vi "CP FES Thresholding.vi"(3 "CP FES Walking Data":T1={"Subject"=0, "Subject Parameter File"=path "", "Subject Parameters"={"Subject"=0, "Left GPD Params"={"% Cycle Delay"=75.0, "Min % Cycle LR to ISw "=55.0, "Min % Cycle LR to MSw"=50.0, "Min % Cycle LR to TSw"=75.0, "Max % Cycle ISw to MSw"=10.0, "Min % Cycle TSw to LR"=2.5, "Max % Cycle TSw to LR"=75.0, "LR Min Gyro Z Threshold"=-0.3, "LR Min Gyro Z Width"=230.0, "ISw Peak Threshold"=0.6, "ISw Peak Width"=55.0, "TSw Valley Threshold"=-0.5, "TSw Valley Width (ms)"=55.0, "Max Cycle Time (s)"=1.3, "Mean Computation Window"=10.0, "CP subject?"=FALSE}, "Right GPD Params"={"% Cycle Delay"=75.0, "Min % Cycle LR to ISw "=55.0, "Min % Cycle LR to MSw"=50.0, "Min % Cycle LR to TSw"=75.0, "Max % Cycle ISw to MSw"=10.0, "Min % Cycle TSw to LR"=2.5, "Max % Cycle TSw to LR"=75.0, "LR Min Gyro Z Threshold"=-0.3, "LR Min Gyro Z Width"=230.0, "ISw Peak Threshold"=0.6, "ISw Peak Width"=55.0, "TSw Valley Threshold"=-0.5, "TSw Valley Width (ms)"=55.0, "Max Cycle Time (s)"=1.3, "Mean Computation Window"=10.0, "CP subject?"=FALSE}, "Left Stim Params"={"Stim Pattern Values"=[[enum."Full", enum."Half", enum."Off", enum."Off", enum."Off", enum."Off", enum."Half"], [enum."Full", enum."Off", enum."Off", enum."Off", enum."Off", enum."Half", enum."Half"], [enum."Half", enum."Full", enum."Off", enum."Full", enum."Off", enum."Off", enum."Full"], [enum."Half", enum."Off", enum."Off", enum."Half", enum."Full", enum."Full", enum."Full"], [enum."Off", enum."Full", enum."Half", enum."Half", enum."Off", enum."Off", enum."Off"]], "Pulse Duration"=[20, 200, 200, 200, 200], "Current"=[20, 20, 20, 20, 20]}, "Right Stim Params"={"Stim Pattern Values"=[[enum."Full", enum."Half", enum."Off", enum."Off", enum."Off", enum."Off", enum."Half"], [enum."Full", enum."Off", enum."Off", enum."Off", enum."Off", enum."Half", enum."Half"], [enum."Half", enum."Full", enum."Off", enum."Full", enum."Off", enum."Off", enum."Full"], [enum."Half", enum."Off", enum."Off", enum."Half", enum."Full", enum."Full", enum."Full"], [enum."Off", enum."Full", enum."Half", enum."Half", enum."Off", enum."Off", enum."Off"]], "Pulse Duration"=[200, 200, 200, 200, 200], "Current"=[200, 200, 200, 200, 200]}, "Left Train length"=[300, 300, 300, 300, 300], "Right Train length"=[300, 300, 300, 300, 300]}, "Current Interval Idx"=0, "Protocol"={"Active Interval"=[], "Protocol"=[{"Interval Type"=enum."Walk", "Duration"=20.0, " Mode"=enum."Stim", "Alt Period"=0.0}, {"Interval Type"=enum."Rest", "Duration"=20.0, " Mode"=enum."No Stim", "Alt Period"=0.0}, {"Interval Type"=enum."Walk", "Duration"=20.0, " Mode"=enum."Stim", "Alt Period"=0.0}, {"Interval Type"=enum."Rest", "Duration"=20.0, " Mode"=enum."No Stim", "Alt Period"=0.0}, {"Interval Type"=enum."Walk", "Duration"=20.0, " Mode"=enum."Stim", "Alt Period"=0.0}, {"Interval Type"=enum."Rest", "Duration"=20.0, " Mode"=enum."No Stim", "Alt Period"=0.0}, {"Interval Type"=enum."Walk", "Duration"=20.0, " Mode"=enum."Stim", "Alt Period"=0.0}, {"Interval Type"=enum."Rest", "Duration"=20.0, " Mode"=enum."No Stim", "Alt Period"=0.0}, {"Interval Type"=enum."Walk", "Duration"=20.0, " Mode"=enum."Alternating", "Alt Period"=0.0}]}, "Stim Protocol Log File"=path "", "APDM Init Cluster"={"Log Data"=TRUE, "Gyro Mode"="SIMULATE GYRO", "Left  OPAL ID"=0, "Right OPAL ID"=0, "Access Point ID"=0}, "Stimulators"=[]} {"Subject" items=["Subject 0", "Subject 1", "Subject 2", "Subject 3", "Subject 4", "Subject 5", "Subject 6", "Subject 7", "Subject 8", "Subject 9", "Subject 10", "Subject 11", "Subject 12", "Subject 13", "Subject 14", "Subject 15", "Subject 16", "Subject 17", "Subject 18", "Subject 19", "Subject 20", "Subject 21", "Subject 22", "Subject 23", "Subject 24", "Subject 25", "Subject 26", "Subject 27", "Subject 28", "Subject 29", "Subject 30", "Subject 31", "Subject 32", "Subject 33", "Subject 34", "Subject 35", "Subject 36", "Subject 37", "Subject 38", "Subject 39", "Subject 40"]; "Subject Parameters"."Subject" items=["Subject 0", "Subject 1", "Subject 2", "Subject 3", "Subject 4", "Subject 5", "Subject 6", "Subject 7", "Subject 8", "Subject 9", "Subject 10", "Subject 11", "Subject 12", "Subject 13", "Subject 14", "Subject 15", "Subject 16", "Subject 17", "Subject 18", "Subject 19", "Subject 20", "Subject 21", "Subject 22", "Subject 23", "Subject 24", "Subject 25", "Subject 26", "Subject 27", "Subject 28", "Subject 29", "Subject 30", "Subject 31", "Subject 32", "Subject 33", "Subject 34", "Subject 35", "Subject 36", "Subject 37", "Subject 38", "Subject 39", "Subject 40"]}) -> (1 "CP FES Walking Data Out":T1={"Subject"=0, "Subject Parameter File"=path "", "Subject Parameters"={"Subject"=0, "Left GPD Params"={"% Cycle Delay"=75.0, "Min % Cycle LR to ISw "=55.0, "Min % Cycle LR to MSw"=50.0, "Min % Cycle LR to TSw"=75.0, "Max % Cycle ISw to MSw"=10.0, "Min % Cycle TSw to LR"=2.5, "Max % Cycle TSw to LR"=75.0, "LR Min Gyro Z Threshold"=-0.3, "LR Min Gyro Z Width"=230.0, "ISw Peak Threshold"=0.6, "ISw Peak Width"=55.0, "TSw Valley Threshold"=-0.5, "TSw Valley Width (ms)"=55.0, "Max Cycle Time (s)"=1.3, "Mean Computation Window"=10.0, "CP subject?"=FALSE}, "Right GPD Params"={"% Cycle Delay"=75.0, "Min % Cycle LR to ISw "=55.0, "Min % Cycle LR to MSw"=50.0, "Min % Cycle LR to TSw"=75.0, "Max % Cycle ISw to MSw"=10.0, "Min % Cycle TSw to LR"=2.5, "Max % Cycle TSw to LR"=75.0, "LR Min Gyro Z Threshold"=-0.3, "LR Min Gyro Z Width"=230.0, "ISw Peak Threshold"=0.6, "ISw Peak Width"=55.0, "TSw Valley Threshold"=-0.5, "TSw Valley Width (ms)"=55.0, "Max Cycle Time (s)"=1.3, "Mean Computation Window"=10.0, "CP subject?"=FALSE}, "Left Stim Params"={"Stim Pattern Values"=[[enum."Full", enum."Half", enum."Off", enum."Off", enum."Off", enum."Off", enum."Half"], [enum."Full", enum."Off", enum."Off", enum."Off", enum."Off", enum."Half", enum."Half"], [enum."Half", enum."Full", enum."Off", enum."Full", enum."Off", enum."Off", enum."Full"], [enum."Half", enum."Off", enum."Off", enum."Half", enum."Full", enum."Full", enum."Full"], [enum."Off", enum."Full", enum."Half", enum."Half", enum."Off", enum."Off", enum."Off"]], "Pulse Duration"=[20, 200, 200, 200, 200], "Current"=[20, 20, 20, 20, 20]}, "Right Stim Params"={"Stim Pattern Values"=[[enum."Full", enum."Half", enum."Off", enum."Off", enum."Off", enum."Off", enum."Half"], [enum."Full", enum."Off", enum."Off", enum."Off", enum."Off", enum."Half", enum."Half"], [enum."Half", enum."Full", enum."Off", enum."Full", enum."Off", enum."Off", enum."Full"], [enum."Half", enum."Off", enum."Off", enum."Half", enum."Full", enum."Full", enum."Full"], [enum."Off", enum."Full", enum."Half", enum."Half", enum."Off", enum."Off", enum."Off"]], "Pulse Duration"=[200, 200, 200, 200, 200], "Current"=[200, 200, 200, 200, 200]}, "Left Train length"=[300, 300, 300, 300, 300], "Right Train length"=[300, 300, 300, 300, 300]}, "Current Interval Idx"=0, "Protocol"={"Active Interval"=[], "Protocol"=[{"Interval Type"=enum."Walk", "Duration"=20.0, " Mode"=enum."Stim", "Alt Period"=0.0}, {"Interval Type"=enum."Rest", "Duration"=20.0, " Mode"=enum."No Stim", "Alt Period"=0.0}, {"Interval Type"=enum."Walk", "Duration"=20.0, " Mode"=enum."Stim", "Alt Period"=0.0}, {"Interval Type"=enum."Rest", "Duration"=20.0, " Mode"=enum."No Stim", "Alt Period"=0.0}, {"Interval Type"=enum."Walk", "Duration"=20.0, " Mode"=enum."Stim", "Alt Period"=0.0}, {"Interval Type"=enum."Rest", "Duration"=20.0, " Mode"=enum."No Stim", "Alt Period"=0.0}, {"Interval Type"=enum."Walk", "Duration"=20.0, " Mode"=enum."Stim", "Alt Period"=0.0}, {"Interval Type"=enum."Rest", "Duration"=20.0, " Mode"=enum."No Stim", "Alt Period"=0.0}, {"Interval Type"=enum."Walk", "Duration"=20.0, " Mode"=enum."Alternating", "Alt Period"=0.0}]}, "Stim Protocol Log File"=path "", "APDM Init Cluster"={"Log Data"=TRUE, "Gyro Mode"="SIMULATE GYRO", "Left  OPAL ID"=0, "Right OPAL ID"=0, "Access Point ID"=0}, "Stimulators"=[]} {"Subject" items=["Subject 0", "Subject 1", "Subject 2", "Subject 3", "Subject 4", "Subject 5", "Subject 6", "Subject 7", "Subject 8", "Subject 9", "Subject 10", "Subject 11", "Subject 12", "Subject 13", "Subject 14", "Subject 15", "Subject 16", "Subject 17", "Subject 18", "Subject 19", "Subject 20", "Subject 21", "Subject 22", "Subject 23", "Subject 24", "Subject 25", "Subject 26", "Subject 27", "Subject 28", "Subject 29", "Subject 30", "Subject 31", "Subject 32", "Subject 33", "Subject 34", "Subject 35", "Subject 36", "Subject 37", "Subject 38", "Subject 39", "Subject 40"]; "Subject Parameters"."Subject" items=["Subject 0", "Subject 1", "Subject 2", "Subject 3", "Subject 4", "Subject 5", "Subject 6", "Subject 7", "Subject 8", "Subject 9", "Subject 10", "Subject 11", "Subject 12", "Subject 13", "Subject 14", "Subject 15", "Subject 16", "Subject 17", "Subject 18", "Subject 19", "Subject 20", "Subject 21", "Subject 22", "Subject 23", "Subject 24", "Subject 25", "Subject 26", "Subject 27", "Subject 28", "Subject 29", "Subject 30", "Subject 31", "Subject 32", "Subject 33", "Subject 34", "Subject 35", "Subject 36", "Subject 37", "Subject 38", "Subject 39", "Subject 40"]})   [LabVIEW 2019]
uses:
  Controls/Muscle Group Labels.ctl
  Controls/Gait Phase Names.ctl
  Controls/Stim off-half-ful.ctl
  Version 2/Data Type Defs/Obsolete/Stimulator Controls_obs.ctl
  Version 2/Data Type Defs/Obsolete/Stimulator Init Control_obs.ctl
  Version 2/Data Type Defs/Stim Init Data.ctl
  Controls/CP FES Walking Data.ctl
  Controls/Subject Params.ctl
  Controls/Subject.ctl
  Controls/GPD Side Parameters.ctl
  Controls/Type Defs/Stim Parameters.ctl
  Controls/Protocol Cluster.ctl
  Controls/Interval on-off indicator.ctl
  Controls/Interval Array.ctl
  Controls/Protocol Interval.ctl
  Controls/Stim Interval Mode.ctl
  Controls/APDM Init Cluster.ctl
  Version 2/Data Type Defs/Stimulator.ctl
  Version 2/Data Type Defs/Stim Open Data.ctl
  Version 2/Data Type Defs/Stim Update Data.ctl
  Version 2/Data Type Defs/Pulse Mode (array).ctl
  Version 2/Data Type Defs/Stim Status.ctl
  Controls/Type Defs/Baseline Threshold Params.ctl
  Controls/Stim Current Array.ctl
  Controls/Pulse Duration Array.ctl
  Controls/Type Defs/Fine Tuning Threshold Params.ctl
  Controls/Train Length Array.ctl
panel:
  out "Subject 2":u16(ring) caption="Subject" items=["Subject 0", "Subject 1", "Subject 2", "Subject 3", "Subject 4", "Subject 5", "Subject 6", "Subject 7", "Subject 8", "Subject 9", "Subject 10", "Subject 11", "Subject 12", "Subject 13", "Subject 14", "Subject 15", "Subject 16", "Subject 17", "Subject 18", "Subject 19", "Subject 20", "Subject 21", "Subject 22", "Subject 23", "Subject 24", "Subject 25", "Subject 26", "Subject 27", "Subject 28", "Subject 29", "Subject 30", "Subject 31", "Subject 32", "Subject 33", "Subject 34", "Subject 35", "Subject 36", "Subject 37", "Subject 38", "Subject 39", "Subject 40"]
  out "Subject Parameter File":path=path "Z:/CP FES Walk/2016 CP CODE/Subject_Parameters/40/CP40_stim_params"
  in  "Tab Control":T19(tab)
  in  "Edit Right Stim Pattern":bool
  in  "Edit Left Stim Pattern":bool
  out "Stim Pattern Display":T22={"_"=["Muscle Groups", "Gluteals", "Hamstrings", "Quadriceps", "Tibialis Anterior", "Triceps Surae"], "Left Stim Pattern"={"Gait Phase Labels  "=["LR", "MSt", "TSt", "PSw", "ISw", "MSw", "TSw"], "Stim Pattern Array"=[]}, "Right Stim Pattern"={"Gait Phase Labels  "=["LR", "MSt", "TSt", "PSw", "ISw", "MSw", "TSw"], "Stim Pattern Array"=[]}}
  out "Right Stim Params":T23={"Pulse Width"=[195, 20, 20, 20, 20, 0, 0, 0, 0, 0], "Current"=[74, 0, 0, 0, 0, 0, 0, 0, 0, 0], "Train length"=[200, 200, 200, 200, 200, 114, 214, 314, 414, 514]} caption="Right Stim Parameters" {"Train length" min=20 max=500 step=5}
  out "Left Stim Params":T23={"Pulse Width"=[195, 20, 20, 20, 20, 0, 0, 0, 0, 0], "Current"=[74, 0, 0, 0, 0, 0, 0, 0, 0, 0], "Train length"=[200, 200, 200, 200, 200, 114, 214, 314, 414, 514]} caption="Left Stim Parameters" {"Train length" min=20 max=500 step=5}
  in  "Left Stim BL":bool
  in  "Left Stim FT":bool
  in  "Right Stim BL":bool
  in  "Right Stim FT":bool
  out "Stimulator Controls":T24={"Stimulator Init Control"={"Stimulator Control"={"Name"="", "Mode"=enum."LIVE", "Visa Timeout"=0}, "Initialization Parameters"={"Stimulator Control"={"Name"="", "Mode"=enum."SIM", "Visa Timeout"=0}, "Initialization Parameters"={"Frequency"=0.0, "N Factor"=0, "D/T Int"=0.0, "Active Channels"=[], "LF Channels"=[]}}}, "Open"=FALSE, "On"=FALSE}
  out "Stim Pattern Control":T26={"_"={"Array 3"=["Muscle Groups"], "Array 2"=["Gluteals", "Hamstrings", "Quadriceps", "Tibialis Anterior", "Triceps Surae"]}, "Left Stim Pattern"={"Gait Phases  "=["LR", "MSt", "TSt", "PSw", "ISw", "MSw", "TSw"], "Left Stim Pattern Values"=[[enum."Full", enum."Half", enum."Off", enum."Off", enum."Off", enum."Off", enum."Half"], [enum."Full", enum."Off", enum."Off", enum."Off", enum."Off", enum."Half", enum."Half"], [enum."Half", enum."Full", enum."Off", enum."Full", enum."Off", enum."Off", enum."Full"], [enum."Half", enum."Off", enum."Off", enum."Half", enum."Full", enum."Full", enum."Full"], [enum."Off", enum."Full", enum."Half", enum."Half", enum."Off", enum."Off", enum."Off"]]}, "Right Stim Pattern"={"Gait Phases  "=["LR", "MSt", "TSt", "PSw", "ISw", "MSw", "TSw"], "Right Stim Pattern Values"=[[enum."Full", enum."Half", enum."Off", enum."Off", enum."Off", enum."Off", enum."Half"], [enum."Full", enum."Off", enum."Off", enum."Off", enum."Off", enum."Half", enum."Half"], [enum."Half", enum."Full", enum."Off", enum."Full", enum."Off", enum."Off", enum."Full"], [enum."Half", enum."Off", enum."Off", enum."Half", enum."Full", enum."Full", enum."Full"], [enum."Off", enum."Full", enum."Half", enum."Half", enum."Off", enum."Off", enum."Off"]]}}
  in  "Reload Parameters":bool
  in  "Done":bool
  # "Add \"all on/all off\""
  # "Gluteals"
  # "Gluteals"
  # "Hamstrings"
  # "Hamstrings"
  # "Quads"
  # "Quads"
  # "TA/Dorsi"
  # "TA/Dorsi"
  # "TS/Plantar"
  # "TS/Plantar"
  # "FOR ADVANCED USERS ONLY"
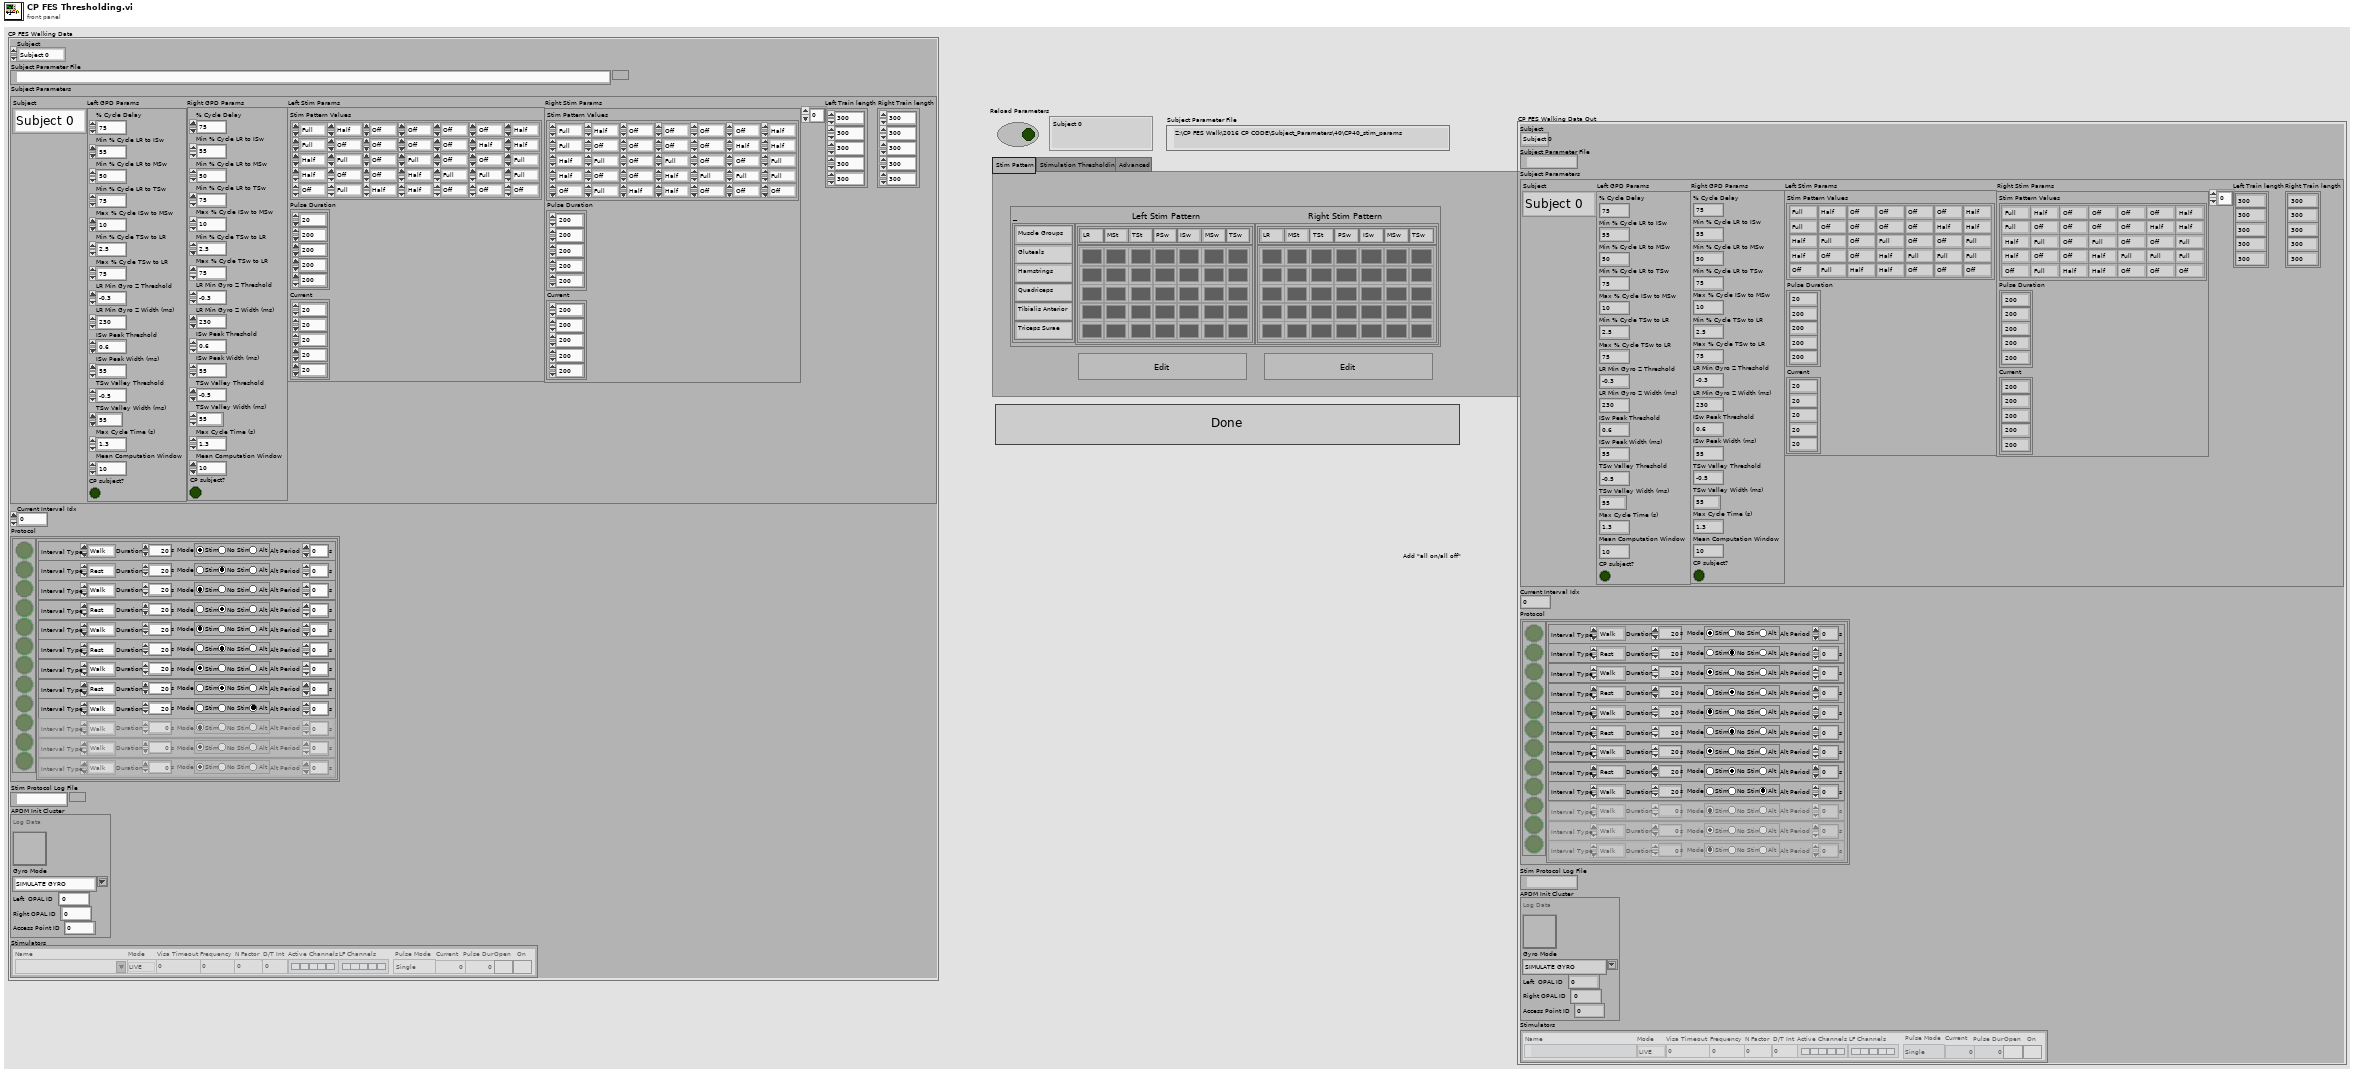
[diagram p1: front panel]
types:
  T1 = typedef "CP FES Walking Data.ctl" = cluster{"Subject":u16, "Subject Parameter File":path, "Subject Parameters":T2, "Current Interval Idx":i32, "Protocol":T7, "Stim Protocol Log File":path, "APDM Init Cluster":T12, "Stimulators":T13[]}
  T2 = typedef "Subject Params.ctl" = cluster{"Subject":T3, "Left GPD Params":T4, "Right GPD Params":T4, "Left Stim Params":T5, "Right Stim Params":T5, "Left Train length":i64[], "Right Train length":i64[]}
  T3 = typedef "Subject.ctl" = u16
  T4 = typedef "GPD Side Parameters.ctl" = cluster{"% Cycle Delay":dbl, "Min % Cycle LR to ISw ":dbl, "Min % Cycle LR to MSw":dbl, "Min % Cycle LR to TSw":dbl, "Max % Cycle ISw to MSw":dbl, "Min % Cycle TSw to LR":dbl, "Max % Cycle TSw to LR":dbl, "LR Min Gyro Z Threshold":dbl, "LR Min Gyro Z Width":dbl, "ISw Peak Threshold":dbl, "ISw Peak Width":dbl, "TSw Valley Threshold":dbl, "TSw Valley Width (ms)":dbl, "Max Cycle Time (s)":dbl, "Mean Computation Window":dbl, "CP subject?":bool}
  T5 = typedef "Stim Parameters.ctl" = cluster{"Stim Pattern Values":T6[][], "Pulse Duration":i64[], "Current":i64[]}
  T6 = typedef "Stim off-half-ful.ctl" = enum16{"Off", "Half", "Full"}
  T7 = typedef "Protocol Cluster.ctl" = cluster{"Active Interval":T8[], "Protocol":T9}
  T8 = typedef "Interval on-off indicator.ctl" = bool
  T9 = typedef "Interval Array.ctl" = T10[]
  T10 = typedef "Protocol Interval.ctl" = cluster{"Interval Type":enum16{"Walk", "Rest"}, "Duration":dbl[unit], " Mode":T11, "Alt Period":dbl[unit]}
  T11 = typedef "Stim Interval Mode.ctl" = enum32{"Stim", "No Stim", "Alternating"}
  T12 = typedef "APDM Init Cluster.ctl" = cluster{"Log Data":bool, "Gyro Mode":string, "Left  OPAL ID":u32, "Right OPAL ID":u32, "Access Point ID":u32}
  T13 = typedef "Stimulator.ctl" = cluster{"Stim Open Data":T14, "Stim Init Data":T15, "Stim Update Data":T16, "Stim Status":T18}
  T14 = typedef "Stim Open Data.ctl" = cluster{"Name":refnum<visa-resource-name>, "Mode":enum16{"LIVE", "SIM"}, "Visa Timeout":u32}
  T15 = typedef "Stim Init Data.ctl" = cluster{"Frequency":dbl, "N Factor":u8, "D/T Int":dbl, "Active Channels":bool[], "LF Channels":bool[]}
  T16 = typedef "Stim Update Data.ctl" = cluster{"Pulse Mode":T17, "Current":u32[], "Pulse Dur":u32[]}
  T17 = typedef "Pulse Mode (array).ctl" = enum16{"Single", "Doublet", "Triplet"}[]
  T18 = typedef "Stim Status.ctl" = cluster{"Open":bool, "On":bool}
  T19 = enum32{"Stim Pattern", "Stimulation Thresholding", "Advanced"}
  T20 = typedef "Muscle Group Labels.ctl" = string[]
  T21 = typedef "Gait Phase Names.ctl" = string[]
  T22 = cluster{"_":T20, "Left Stim Pattern":cluster{"Gait Phase Labels  ":T21, "Stim Pattern Array":u32[][]}, "Right Stim Pattern":cluster{"Gait Phase Labels  ":T21, "Stim Pattern Array":u32[][]}}
  T23 = cluster{"Pulse Width":i64[], "Current":i64[], "Train length":i64[]}
  T24 = typedef "Stimulator Controls_obs.ctl" = cluster{"Stimulator Init Control":cluster{"Stimulator Control":cluster{"Name":refnum<visa-resource-name>, "Mode":enum16{"LIVE", "SIM"}, "Visa Timeout":u32}, "Initialization Parameters":T25}, "Open":bool, "On":bool}
  T25 = typedef "Stimulator Init Control_obs.ctl" = cluster{"Stimulator Control":cluster{"Name":refnum<visa-resource-name>, "Mode":enum16{"LIVE", "SIM"}, "Visa Timeout":u32}, "Initialization Parameters":T15}
  T26 = cluster{"_":cluster{"Array 3":string[], "Array 2":string[]}, "Left Stim Pattern":cluster{"Gait Phases  ":T21, "Left Stim Pattern Values":T6[][]}, "Right Stim Pattern":cluster{"Gait Phases  ":T21, "Right Stim Pattern Values":T6[][]}}
  T27 = typedef "Baseline Threshold Params.ctl" = cluster{"Current":T28, "Pulse Duration":T29}
  T28 = typedef "Stim Current Array.ctl" = u8[]
  T29 = typedef "Pulse Duration Array.ctl" = u32[]
  T30 = typedef "Fine Tuning Threshold Params.ctl" = cluster{"Current":T28, "Pulse Duration":T29, "Train Length":T31}
  T31 = typedef "Train Length Array.ctl" = i64[]
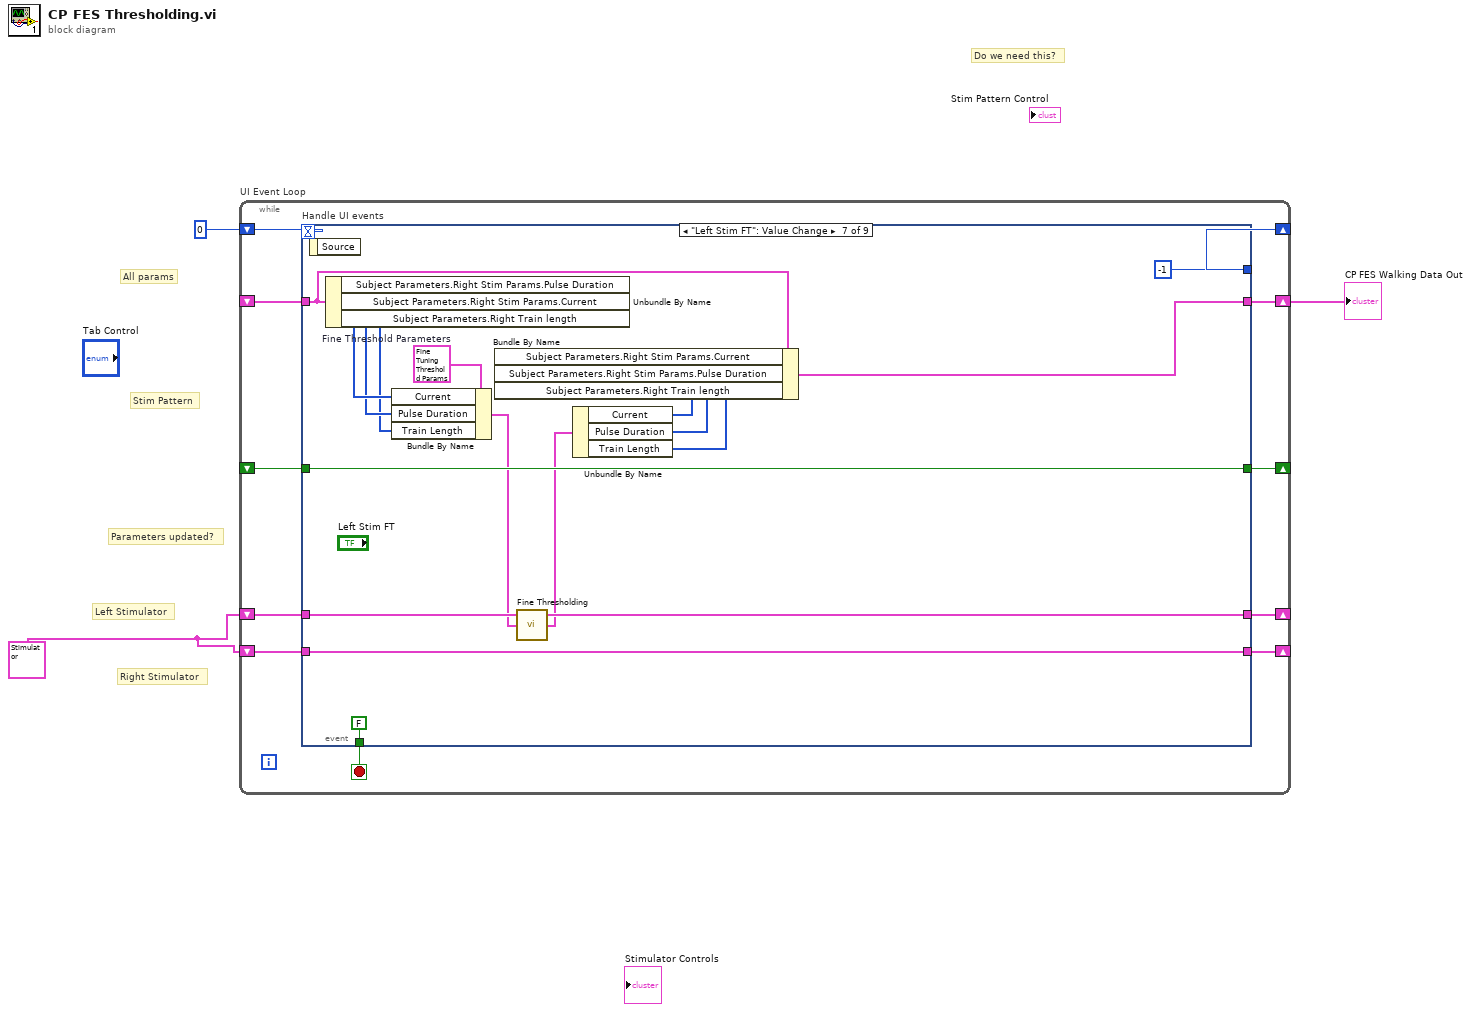
[diagram p0: block diagram]
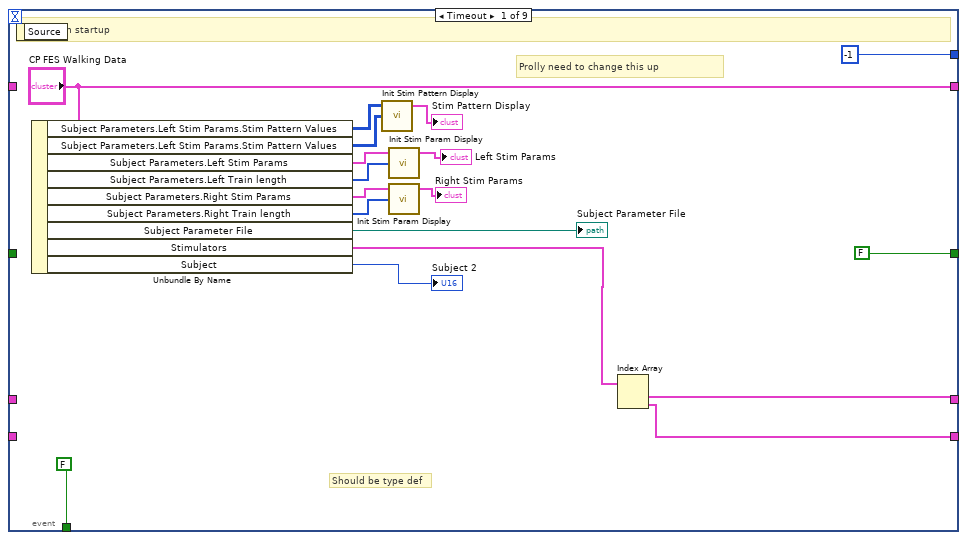
[diagram p2: hidden frame]
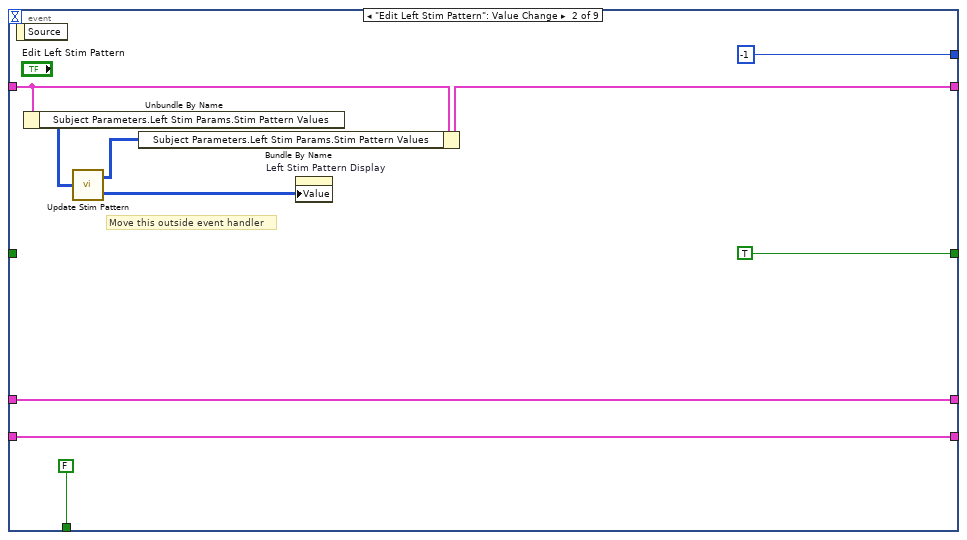
[diagram p3: hidden frame]
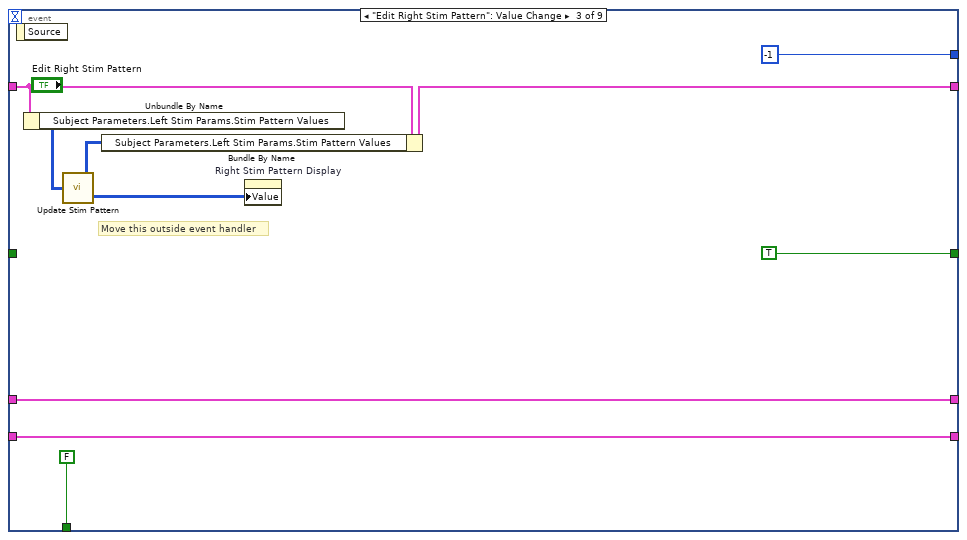
[diagram p4: hidden frame]
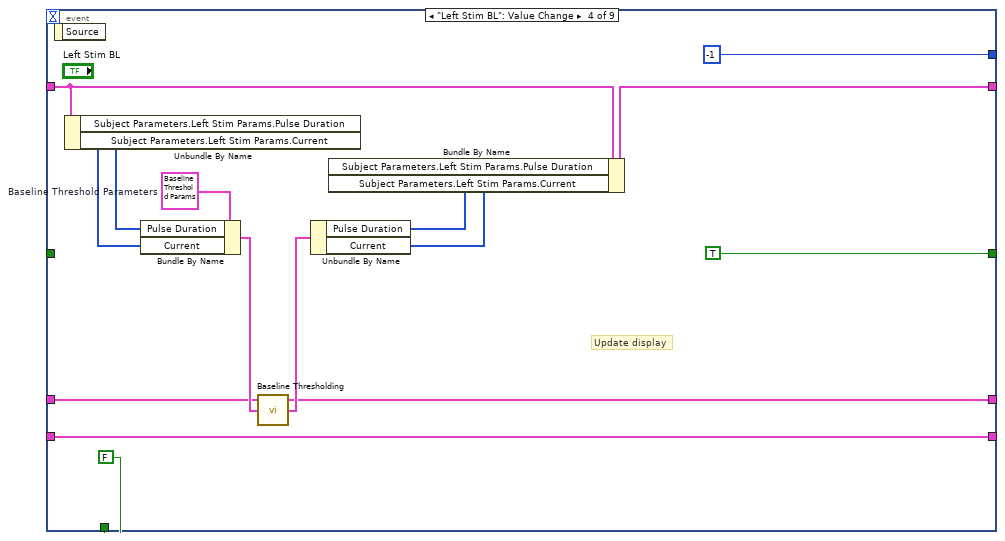
[diagram p5: hidden frame]
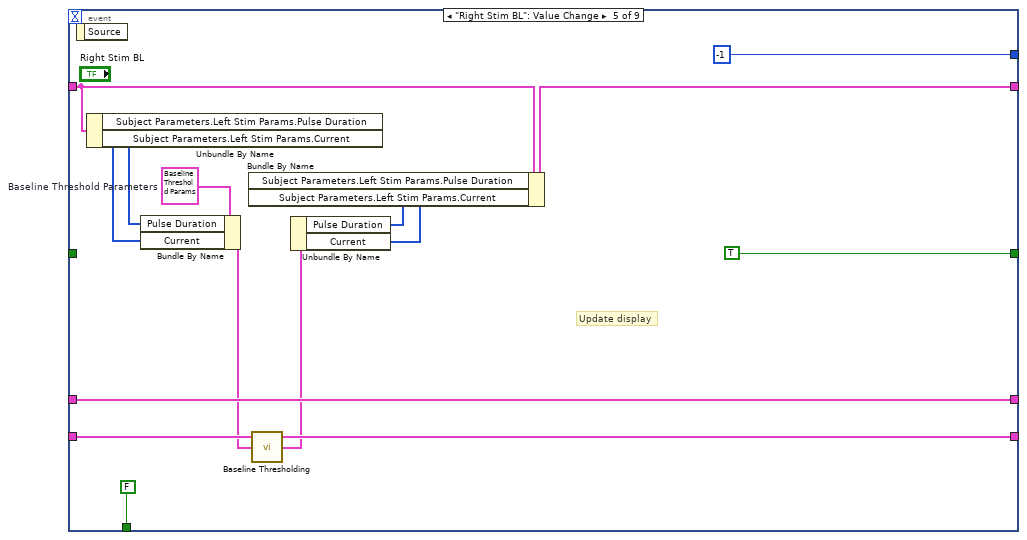
[diagram p6: hidden frame]
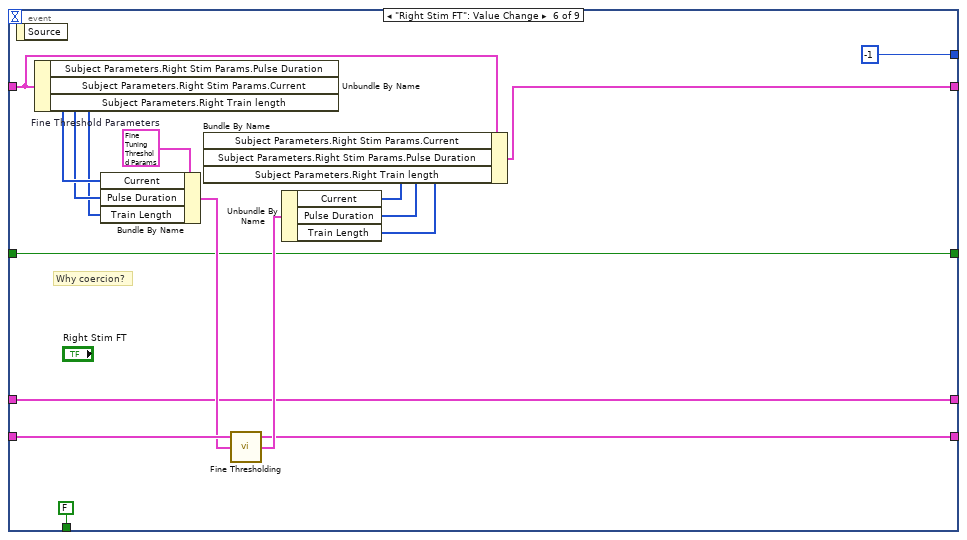
[diagram p7: hidden frame]
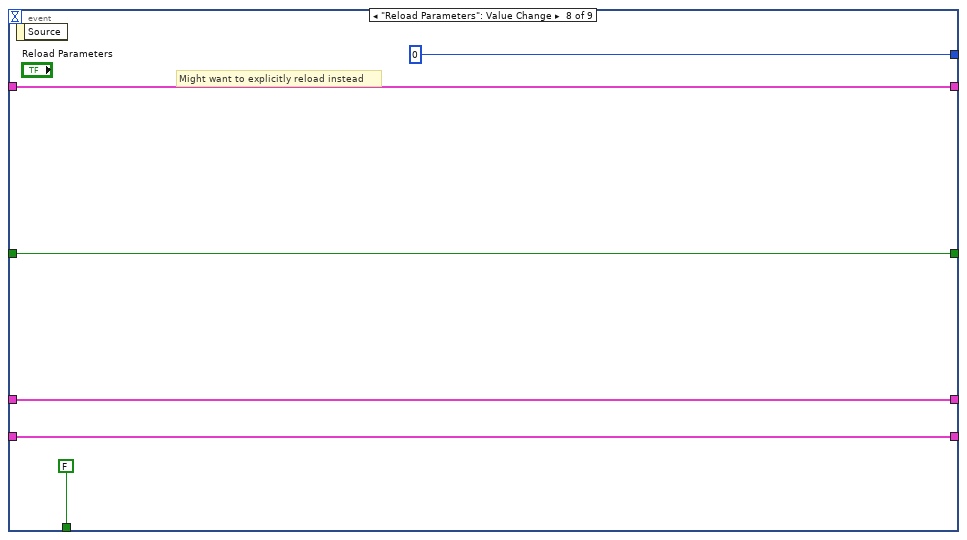
[diagram p8: hidden frame]
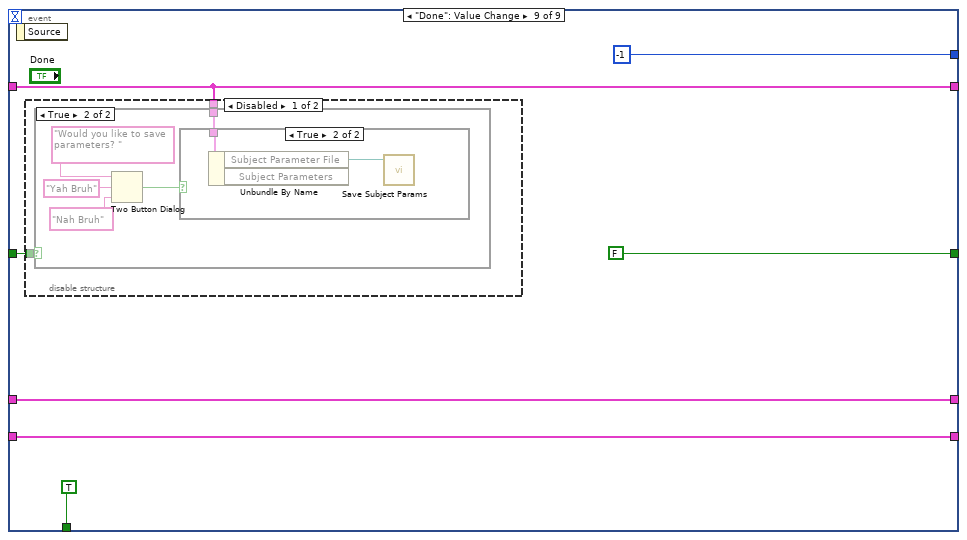
[diagram p9: hidden frame]
diagram:
  w1 = T13 {"Stim Open Data"={"Name"="", "Mode"=enum."LIVE", "Visa Timeout"=0}, "Stim Init Data"={"Frequency"=0.0, "N Factor"=0, "D/T Int"=0.0, "Active Channels"=[], "LF Channels"=[]}, "Stim Update Data"={"Pulse Mode"=[enum."Single"], "Current"=[], "Pulse Dur"=[]}, "Stim Status"={"Open"=FALSE, "On"=FALSE}} ("element")
  # "Do we need this?"
  # "All params"
  # "Stim Pattern"
  # "Right Stimulator"
  # "Left Stimulator"
  # "Parameters updated?"
  n1 = while "UI Event Loop" {
    shift-right: [w11] -> _
    shift-left: 0 -> [w13]
    shift-right: [w7] -> _
    shift-left: w1 -> [w5]
    shift-right: [w6] -> _
    shift-left: w1 -> [w4]
    shift-right: [w10] -> _
    shift-left: _ -> [w12]
    shift-right: [w8] -> w2
    shift-left: _ -> [w9]
    stop <- w14 stop-if-true
    n2 = event "Handle UI events" shown="[6] \"Left Stim FT\": Value Change" {
      selector: _ -> [_ _ _ _ _ _ _ _ _]
      dyn-events: _ -> [_ _ _ _ _ _ _ _ _]
      timeout: w13 -> [_ _ _ _ _ _ _ _ _]
      tunnel: [FALSE ("Done") FALSE ("Done") FALSE ("Done") FALSE ("Done") FALSE ("Done") FALSE ("Done") FALSE ("Done") FALSE TRUE ("Done")] -> w14
      tunnel: [w15 w39 w49 w66 w80 w83 w105 w118 w125] -> w6
      tunnel: [w16 w40 w50 w53 w79 w85 w103 w119 w126] -> w7
      tunnel: w4 -> [_ w39 w49 w66 w81 w95 w105 w118 w125]
      tunnel: w5 -> [_ w40 w50 w54 w79 w85 w104 w119 w126]
      tunnel: [FALSE TRUE TRUE TRUE TRUE w86 w106 w120 FALSE] -> w10
      tunnel: w12 -> [_ _ _ _ _ w86 w106 w120 w127]
      tunnel: [-1 -1 -1 -1 -1 -1 -1 0 -1] -> w11
      tunnel: ["CP FES Walking Data" w34 w43 w60 w68 w88 w108 w117 w124] -> w8
      tunnel: w9 -> [_ w35 w44 w61 w69 w93 w109 w117 w124]
      event Timeout {
        # "Prolly need to change this up"
        # "Should be type def"
        # "Execute on startup"
        n3 = event-data() -> ()  [unwired: 1 in, 1 out]
        n4 = Unbundle By Name("CP FES Walking Data") -> ("Subject Parameters.Left Stim Params.Stim Pattern Values"=w31:T6[][], "Subject Parameters.Left Stim Params.Stim Pattern Values"=w30:T6[][], "Subject Parameters.Left Stim Params"=w26:T5, "Subject Parameters.Left Train length"=w24:i64[], "Subject Parameters.Right Stim Params"=w23:T5, "Subject Parameters.Right Train length"=w22:i64[], "Subject Parameter File"=→"Subject Parameter File":path, "Stimulators"=w17:T13[], "Subject"=→"Subject 2":u16)
        n5 = call "Init Stim Pattern Display.vi"("Stim Pattern Values"=w30, "Stim Pattern Values 2"=w31) -> ("Stim Pattern Display"=→"Stim Pattern Display":T22)  [unwired: 3 in]
        n6 = call "Init Stim Param Display.vi"("Left Train length"=w24, "Left Stim Params in"=w26) -> ("Left Stim Params out"=→"Left Stim Params":T23)  [unwired: 3 in]
        n7 = call "Init Stim Param Display.vi"("Left Train length"=w22, "Left Stim Params in"=w23) -> ("Left Stim Params out"=→"Right Stim Params":T23)  [unwired: 3 in]
        n8 = Index Array(array=w17) -> (element #1=w16:T13, element #2=w15:T13)  [unwired: 2 in]
      }
      event "Edit Left Stim Pattern": Value Change {
        # "Move this outside event handler"
        n9 = event-data() -> ()  [unwired: 1 in, 1 out]
        n10 = Unbundle By Name(w35) -> ("Subject Parameters.Left Stim Params.Stim Pattern Values"=w37:T6[][])
        n11 = call "Update Stim Pattern.vi"("Stim Pattern In"=w37) -> ("Stim Pattern Out"=w36:T6[][], "Pretty Colors Out"=w33:u32[][])
        n12 = Bundle By Name(cluster=w35, "Subject Parameters.Left Stim Params.Stim Pattern Values"=w36) -> (w34:T1)
        n13 = property on="Left Stim Pattern Display" class="Arr (strict)"("Value"=w33) -> ()  [unwired: 2 in, 2 out]
      }
      event "Edit Right Stim Pattern": Value Change {
        # "Move this outside event handler"
        n14 = event-data() -> ()  [unwired: 1 in, 1 out]
        n15 = Unbundle By Name(w44) -> ("Subject Parameters.Left Stim Params.Stim Pattern Values"=w47:T6[][])
        n16 = call "Update Stim Pattern.vi"("Stim Pattern In"=w47) -> ("Stim Pattern Out"=w46:T6[][], "Pretty Colors Out"=w45:u32[][])
        n17 = Bundle By Name(cluster=w44, "Subject Parameters.Left Stim Params.Stim Pattern Values"=w46) -> (w43:T1)
        n18 = property on="Right Stim Pattern Display" class="Arr (strict)"("Value"=w45) -> ()  [unwired: 2 in, 2 out]
      }
      event "Left Stim BL": Value Change {
        w59 = T27 {"Current"=[20, 20, 20, 20, 20], "Pulse Duration"=[500, 500, 500, 500]}  # Baseline Threshold Parameters
        # "Update display"
        n19 = event-data() -> ()  [unwired: 1 in, 1 out]
        n20 = Unbundle By Name(w61) -> ("Subject Parameters.Left Stim Params.Pulse Duration"=w63:i64[], "Subject Parameters.Left Stim Params.Current"=w62:i64[])
        n21 = Bundle By Name(cluster=w59, "Pulse Duration"=w63, "Current"=w62) -> (w58:T27)
        n22 = call "Baseline Thresholding.vi"("Baseline Threshold Parameters"=w58, "Stimulator"=w54) -> ("Baseline Threshold Params Out"=w57:T27, "Stimulator Out"=w53:T13)  [unwired: 2 in]
        n23 = Unbundle By Name(w57) -> ("Pulse Duration"=w56:T29, "Current"=w55:T28)
        n24 = Bundle By Name(cluster=w61, "Subject Parameters.Left Stim Params.Pulse Duration"=w56, "Subject Parameters.Left Stim Params.Current"=w55) -> (w60:T1)
      }
      event "Right Stim BL": Value Change {
        w74 = T27 {"Current"=[20, 20, 20, 20, 20], "Pulse Duration"=[500, 500, 500, 500]}  # Baseline Threshold Parameters
        # "Update display"
        n25 = event-data() -> ()  [unwired: 1 in, 1 out]
        n26 = Unbundle By Name(w69) -> ("Subject Parameters.Left Stim Params.Pulse Duration"=w76:i64[], "Subject Parameters.Left Stim Params.Current"=w75:i64[])
        n27 = Bundle By Name(cluster=w74, "Pulse Duration"=w76, "Current"=w75) -> (w73:T27)
        n28 = call "Baseline Thresholding.vi"("Baseline Threshold Parameters"=w73, "Stimulator"=w81) -> ("Baseline Threshold Params Out"=w72:T27, "Stimulator Out"=w80:T13)  [unwired: 2 in]
        n29 = Unbundle By Name(w72) -> ("Pulse Duration"=w71:T29, "Current"=w70:T28)
        n30 = Bundle By Name(cluster=w69, "Subject Parameters.Left Stim Params.Pulse Duration"=w71, "Subject Parameters.Left Stim Params.Current"=w70) -> (w68:T1)
      }
      event "Right Stim FT": Value Change {
        w99 = T30 {"Current"=[20, 20, 20, 20, 20], "Pulse Duration"=[500, 500, 500, 500], "Train Length"=[200, 200, 200, 200, 200, 114, 214, 314, 414, 514]}  # Fine Threshold Parameters
        # "Why coercion?"
        n31 = event-data() -> ()  [unwired: 1 in, 1 out]
        n32 = Unbundle By Name(w93) -> ("Subject Parameters.Right Stim Params.Pulse Duration"=w98:i64[], "Subject Parameters.Right Stim Params.Current"=w97:i64[], "Subject Parameters.Right Train length"=w96:i64[])
        n33 = Bundle By Name(cluster=w99, "Current"=w98, "Pulse Duration"=w97, "Train Length"=w96) -> (w94:T30)
        n34 = call "Fine Thresholding.vi"("Fine Threshold Parameters"=w94, "Stimulator"=w95) -> ("Fine Threshold Parameters"=w92:T30, "Stimulator"=w83:T13)  [unwired: 2 in]
        n35 = Unbundle By Name(w92) -> ("Current"=w91:T28, "Pulse Duration"=w90:T29, "Train Length"=w89:T31)
        n36 = Bundle By Name(cluster=w93, "Subject Parameters.Right Stim Params.Current"=w91, "Subject Parameters.Right Stim Params.Pulse Duration"=w90, "Subject Parameters.Right Train length"=w89) -> (w88:T1)
      }
      event "Left Stim FT": Value Change {
        w116 = T30 {"Current"=[20, 20, 20, 20, 20], "Pulse Duration"=[500, 500, 500, 500], "Train Length"=[200, 200, 200, 200, 200, 114, 214, 314, 414, 514]}  # Fine Threshold Parameters
        n37 = event-data() -> ()  [unwired: 1 in, 1 out]
        n38 = Unbundle By Name(w109) -> ("Subject Parameters.Right Stim Params.Pulse Duration"=w115:i64[], "Subject Parameters.Right Stim Params.Current"=w114:i64[], "Subject Parameters.Right Train length"=w113:i64[])
        n39 = Bundle By Name(cluster=w116, "Current"=w115, "Pulse Duration"=w114, "Train Length"=w113) -> (w102:T30)
        n40 = call "Fine Thresholding.vi"("Fine Threshold Parameters"=w102, "Stimulator"=w104) -> ("Fine Threshold Parameters"=w101:T30, "Stimulator"=w103:T13)  [unwired: 2 in]
        n41 = Unbundle By Name(w101) -> ("Current"=w112:T28, "Pulse Duration"=w111:T29, "Train Length"=w110:T31)
        n42 = Bundle By Name(cluster=w109, "Subject Parameters.Right Stim Params.Current"=w112, "Subject Parameters.Right Stim Params.Pulse Duration"=w111, "Subject Parameters.Right Train length"=w110) -> (w108:T1)
      }
      event "Reload Parameters": Value Change {
        # "Might want to explicitly reload instead"
        n43 = event-data() -> ()  [unwired: 1 in, 1 out]
      }
      event "Done": Value Change {
        n44 = event-data() -> ()  [unwired: 1 in, 1 out]
        n45 = disable-structure shown="Disabled" {
          disable-tunnel: w127 -> [w131 _]
          disable-tunnel: w124 -> [w130 _]
          frame Disabled {
            n46 = case shown="True" w131 {
              tunnel: w130 -> [_ w132]
              frame False {
              }
              frame True {
                n47 = Two Button Dialog(message="Would you like to save parameters? ", 1:"Nah Bruh" ("F button name (\"Cancel\")"), 2:"Yah Bruh" ("T button name (\"OK\")")) -> (T button?=w133:bool)
                n48 = case shown="True" w133 {
                  tunnel: w132 -> [_ w138]
                  frame False {
                  }
                  frame True {
                    n49 = Unbundle By Name(w138) -> ("Subject Parameter File"=w137:path)  [unwired: 1 out]
                    n50 = call "Save Subject Params.vi"("Subject Parameters File"=w137) -> ()  [unwired: 4 in, 1 out]
                  }
                }
              }
            }
          }
          frame Enabled {
          }
        }
      }
    }
  }
  "CP FES Walking Data Out" <- w2
